vi "String to Timestamp.vi"(10 "Timestamp String":string) -> (2 "Timestamp":timestamp)   [LabVIEW 2020, in "IniFileSection.lvclass"]
uses:
  <vilib>/gpm_packages/@cs/Configuration/Source/IniFileSection/IniFileSection.lvclass
  <vilib>/Utility/miscctls.llb/LVDateTimeRec.ctl
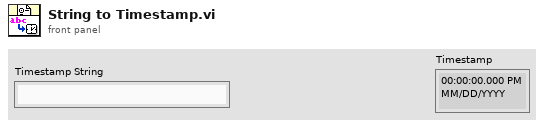
[diagram p1: front panel]
types:
  T1 = typedef "LVDateTimeRec.ctl" = cluster{"fractional second":dbl, "second":i32, "minute":i32, "hour":i32, "day of month":i32, "month":i32, "year":i32, "day of week":i32, "day of year":i32, "DST":i32}
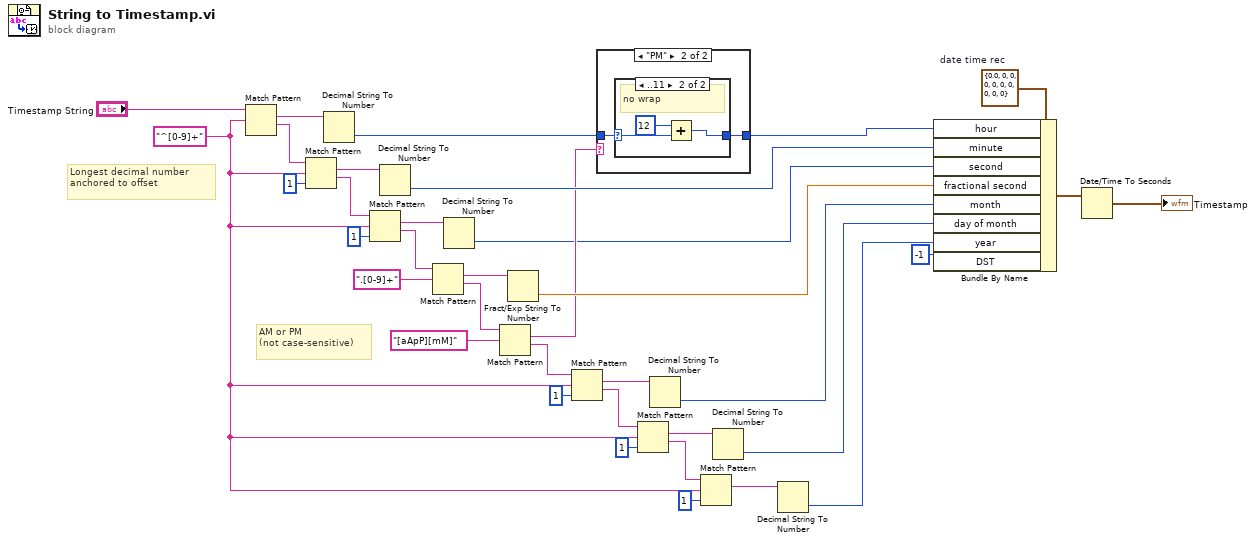
[diagram p0: block diagram]
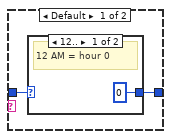
[diagram p2: hidden frame]
diagram:
  w6 = "^[0-9]+" ("Regex")
  w36 = T1 {"fractional second"=0.0, "second"=0, "minute"=0, "hour"=0, "day of month"=0, "month"=0, "year"=0, "day of week"=0, "day of year"=0, "DST"=0}  # date time rec
  # "AM or PM\n(not case-sensitive)"
  # "Longest decimal number\nanchored to offset"
  n1 = Match Pattern(string="Timestamp String", regular expression=w6) -> (match substring=w34:string, after substring=w32:string)  [unwired: 1 in, 2 out]
  n2 = Match Pattern(string=w32, regular expression=w6, offset (0)=1) -> (match substring=w31:string, after substring=w30:string)  [unwired: 2 out]
  n3 = Decimal String To Number(string=w34) -> (number=w19:i32)  [unwired: 2 in, 1 out]
  n4 = Match Pattern(string=w30, regular expression=w6, offset (0)=1) -> (match substring=w29:string, after substring=w26:string)  [unwired: 2 out]
  n5 = Decimal String To Number(string=w31) -> (number=w33:i32)  [unwired: 2 in, 1 out]
  n6 = Match Pattern(string=w26, regular expression=".[0-9]+") -> (match substring=w24:string, after substring=w22:string)  [unwired: 1 in, 2 out]
  n7 = Decimal String To Number(string=w29) -> (number=w10:i32)  [unwired: 2 in, 1 out]
  n8 = Match Pattern(string=w22, regular expression="[aApP][mM]") -> (match substring=w20:string, after substring=w11:string)  [unwired: 1 in, 2 out]
  n9 = Fract/Exp String To Number(string=w24) -> (number=w23:dbl)  [unwired: 3 in, 1 out]
  n10 = Match Pattern(string=w11, regular expression=w6, offset (0)=1) -> (match substring=w17:string, after substring=w13:string)  [unwired: 2 out]
  n11 = case shown="\"PM\"" w20 {
    tunnel: w19 -> [w38 w42]
    tunnel: [w37 w41] -> w18
    frame Default {
      n12 = case shown="12.." w38 {
        selector: w38 -> [_ w40]
        tunnel: [0 w40] -> w37
        frame 12.. {
          # "12 AM = hour 0"
        }
        frame ..11 {
          # "no wrap"
        }
      }
    }
    frame "PM" {
      n13 = case shown="..11" w42 {
        selector: w42 -> [w43 w46]
        tunnel: [w43 w45] -> w41
        frame 12.. {
          # "12 PM --> +0"
        }
        frame ..11 {
          # "no wrap"
          n14 = Add(x=12, y=w46) -> (x+y=w45:i32)
        }
      }
    }
  }
  n15 = Match Pattern(string=w13, regular expression=w6, offset (0)=1) -> (match substring=w15:string, after substring=w12:string)  [unwired: 2 out]
  n16 = Decimal String To Number(string=w17) -> (number=w16:i32)  [unwired: 2 in, 1 out]
  n17 = Match Pattern(string=w12, regular expression=w6, offset (0)=1) -> (match substring=w14:string)  [unwired: 3 out]
  n18 = Decimal String To Number(string=w15) -> (number=w9:i32)  [unwired: 2 in, 1 out]
  n19 = Decimal String To Number(string=w14) -> (number=w8:i32)  [unwired: 2 in, 1 out]
  n20 = Bundle By Name(cluster=w36, "hour"=w18, "minute"=w33, "second"=w10, "fractional second"=w23, "month"=w16, "day of month"=w9, "year"=w8, "DST"=-1) -> (w35:T1)
  n21 = Date/Time To Seconds(2:w35) -> (0:→"Timestamp":timestamp)  [unwired: 1 in]
